vi "Paths.vi"() -> (0 "ppl Path":path, 1 "cfg Path":path, 2 "bin Path":path, 3 "App.Kind":string)   [LabVIEW 2020, in "neg-pkg.lvlib"]
uses:
  neg-pkg.lvlib
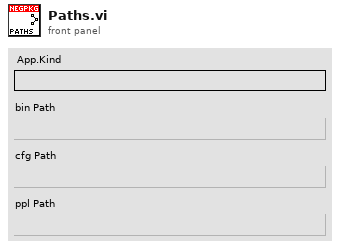
[diagram p1: front panel]
types:
  T1 = enum32{"invalid app kind", "Development System", "Run Time System", "Student Edition", "Embedded LabVIEW", "Evaluation", "Custom", "Community Edition"}
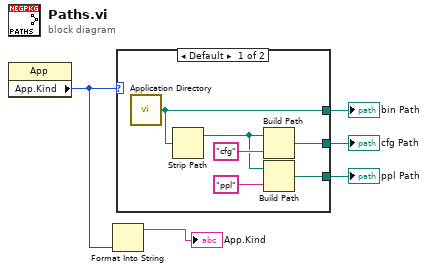
[diagram p0: block diagram]
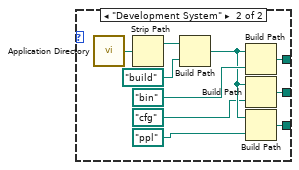
[diagram p2: hidden frame]
diagram:
  n1 = property class="App"() -> ("App.Kind"=w2:T1)  [unwired: 2 in, 2 out]
  n2 = Format Into String(w2) -> (resulting string=→"App.Kind":string)  [unwired: 3 in, 1 out]
  n3 = case shown="Default" w2 {
    tunnel: [w7 w21] -> w5
    tunnel: [w9 w20] -> w4
    tunnel: [w8 w19] -> w3
    frame Default {
      n4 = call <vilib>:"Application Directory.vi"() -> ("Application Directory"=w7:path)
      n5 = Strip Path(path=w7) -> (stripped path=w6:path)  [unwired: 1 out]
      n6 = Build Path(base path=w6, name or relative path="cfg") -> (appended path=w9:path)
      n7 = Build Path(base path=w6, name or relative path="ppl") -> (appended path=w8:path)
    }
    frame "Development System" {
      n8 = call <vilib>:"Application Directory.vi"() -> ("Application Directory"=w18:path)
      n9 = Strip Path(path=w18) -> (stripped path=w17:path)  [unwired: 1 out]
      n10 = Build Path(base path=w17, name or relative path=path "build") -> (appended path=w14:path)
      n11 = Build Path(base path=w14, name or relative path=path "bin") -> (appended path=w21:path)
      n12 = Build Path(base path=w14, name or relative path=path "cfg") -> (appended path=w20:path)
      n13 = Build Path(base path=w14, name or relative path=path "ppl") -> (appended path=w19:path)
    }
  }
  "bin Path" <- w5
  "cfg Path" <- w4
  "ppl Path" <- w3
